vi "Configure Continuous Acquisition.vi"(8 "error in (no error)":errorcluster, 10 "Enable Continuous Acquisition (T:Enable)":bool=TRUE, 11 "VISA resource name":refnum<visa-resource-name>) -> (0 "error out":errorcluster, 3 "VISA resource name out":refnum<visa-resource-name>)   [LabVIEW 2015, in "Template - Scope.lvlib"]
doc: "Configures the instrument to run continuously or to stop after a single configured acquisition.\n\n<B>Note:</B>\n(1) This setting does not occur until the Initiate VI or <b>Read Waveform </b>VI is called.\n(2) Performing an Autosetup puts the instrument in continuous acquisition mode."
uses:
  <instrlib>/_Template - Scope/Template - Scope.lvlib
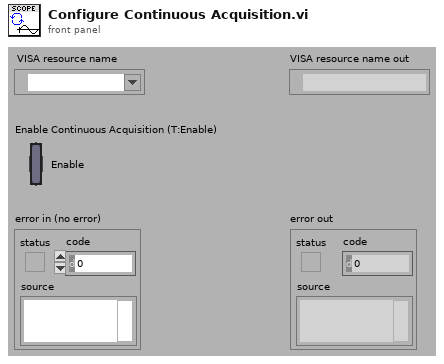
[diagram p1: front panel]
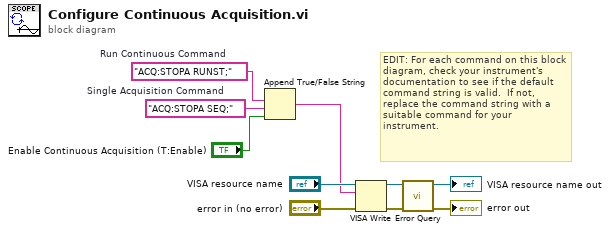
[diagram p0: block diagram]
diagram:
  w3 = "ACQ:STOPA SEQ;"  # Single Acquisition Command
  w4 = "ACQ:STOPA RUNST;"  # Run Continuous Command
  # "EDIT: For each command on this block diagram, check your instrument's documentation to see if the default command string is valid.  If not, replace the command string with a suitable command for your instrument."
  n1 = Append True/False String(1:"Enable Continuous Acquisition (T:Enable)", 2:w3, 3:w4) -> (0:w1:string)  [unwired: 1 in]
  n2 = VISA Write(VISA resource name="VISA resource name", write buffer=w1, error in (no error)="error in (no error)") -> (VISA resource name out=w6:refnum<visa-resource-name>, error out=w5:errorcluster)  [unwired: 1 out]
  n3 = call <instrlib>:"Error Query.vi"("error in (no error)"=w5, "VISA resource name"=w6) -> ("error out"=→"error out":errorcluster, "VISA resource name out"=→"VISA resource name out":refnum<visa-resource-name>)  [unwired: 6 in, 2 out]
